vi "JSON GRUPO 1.vi"(0 "Result":cluster{u32, dbl, dbl, dbl, dbl}[](array[cluster]), 11 "error in":errorcluster) -> (4 "PAR":refnum<class "JSON Object.lvclass">[](array[class]), 6 "Humedad R.":refnum<class "JSON Object.lvclass">[](array[class]), 8 "Temp Amb":refnum<class "JSON Object.lvclass">[](array[class]), 10 "Temp Panel":refnum<class "JSON Object.lvclass">[](array[class]), 15 "error out":errorcluster)   [LabVIEW 2015]
uses:
  <vilib>/addons/JSON API/Get Polymorphic/JSON GetSet.lvlib
  <vilib>/addons/JSON API/JSON Scalar/Set SGL.vi
  <vilib>/addons/JSON API/JSON Scalar/JSON Scalar.lvclass
  <vilib>/addons/JSON API/JSON Scalar/Set U32.vi
  <vilib>/addons/JSON API/JSON Object/Set Object Item by name.vi
  <vilib>/addons/JSON API/JSON Object/JSON Object.lvclass
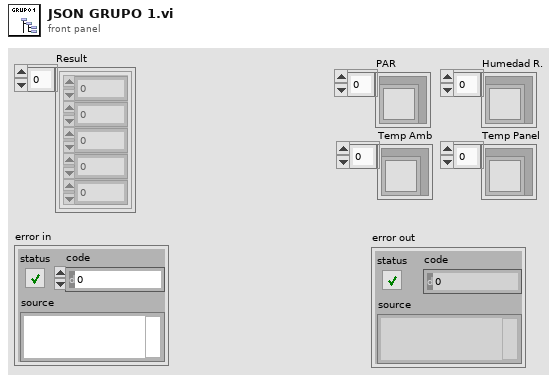
[diagram p1: front panel]
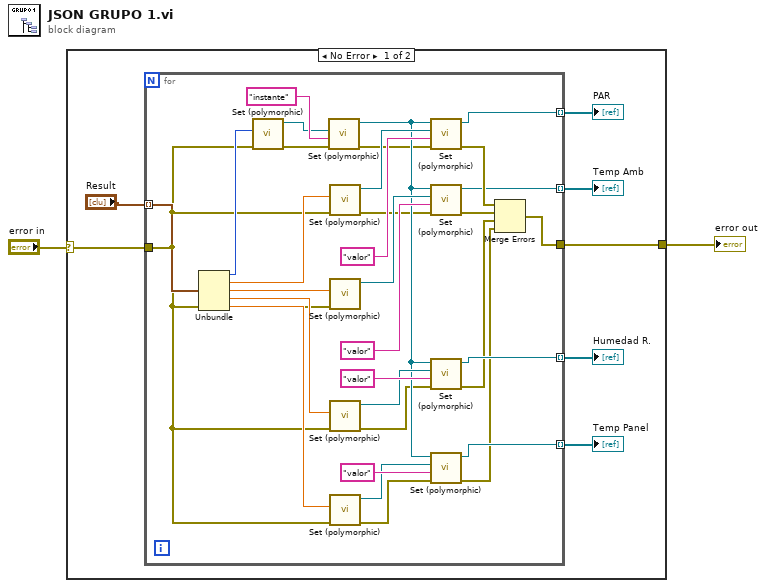
[diagram p0: block diagram]
diagram:
  n1 = case shown="No Error" "error in" {
    selector: "error in" -> [w3 w42]
    tunnel: [w8 w42] -> w1
    frame No Error {
      n2 = for {
        tunnel: "Result" -> [w41] mode=indexing
        tunnel: [w17] -> w7 mode=indexing
        tunnel: [w15] -> w6 mode=indexing
        tunnel: [w13] -> w5 mode=indexing
        tunnel: [w11] -> w4 mode=indexing
        tunnel: w3 -> [w24]
        tunnel: [w18] -> w8
        n3 = Unbundle(w41) -> (w36:u32, w40:dbl, w39:dbl, w38:dbl, w37:dbl)
        n4 = call-poly <vilib>:"Set (polymorphic).vi"("error in (no error)"=w24, "Numeric"=w36) -> ("error out"=w23:errorcluster, "JSON Scalar out"=w34:refnum<class "JSON Scalar.lvclass">)  [unwired: 8 in]
        n5 = call-poly <vilib>:"Set (polymorphic).vi"("error in (no error)"=w23, "name"="instante", "Value"=w34) -> ("error out"=w22:errorcluster, "JSON Object out"=w25:refnum<class "JSON Object.lvclass">)  [unwired: 6 in, 1 out]
        n6 = call-poly <vilib>:"Set (polymorphic).vi"("error in (no error)"=w24, "Numeric"=w40) -> ("error out"=w21:errorcluster, "JSON Scalar out"=w32:refnum<class "JSON Scalar.lvclass">)  [unwired: 8 in]
        n7 = call-poly <vilib>:"Set (polymorphic).vi"("error in (no error)"=w24, "Numeric"=w39) -> ("JSON Scalar out"=w30:refnum<class "JSON Scalar.lvclass">)  [unwired: 8 in, 1 out]
        n8 = call-poly <vilib>:"Set (polymorphic).vi"("error in (no error)"=w24, "Numeric"=w38) -> ("error out"=w20:errorcluster, "JSON Scalar out"=w28:refnum<class "JSON Scalar.lvclass">)  [unwired: 8 in]
        n9 = call-poly <vilib>:"Set (polymorphic).vi"("error in (no error)"=w24, "Numeric"=w37) -> ("error out"=w19:errorcluster, "JSON Scalar out"=w26:refnum<class "JSON Scalar.lvclass">)  [unwired: 8 in]
        n10 = call-poly <vilib>:"Set (polymorphic).vi"("error in (no error)"=w22, "name"="valor", "Value"=w32, "JSON Object in"=w25) -> ("error out"=w16:errorcluster, "JSON Object out"=w17:refnum<class "JSON Object.lvclass">)  [unwired: 5 in, 1 out]
        n11 = call-poly <vilib>:"Set (polymorphic).vi"("error in (no error)"=w21, "name"="valor", "Value"=w30, "JSON Object in"=w25) -> ("error out"=w14:errorcluster, "JSON Object out"=w15:refnum<class "JSON Object.lvclass">)  [unwired: 5 in, 1 out]
        n12 = call-poly <vilib>:"Set (polymorphic).vi"("error in (no error)"=w20, "name"="valor", "Value"=w28, "JSON Object in"=w25) -> ("error out"=w12:errorcluster, "JSON Object out"=w13:refnum<class "JSON Object.lvclass">)  [unwired: 5 in, 1 out]
        n13 = call-poly <vilib>:"Set (polymorphic).vi"("error in (no error)"=w19, "name"="valor", "Value"=w26, "JSON Object in"=w25) -> ("error out"=w10:errorcluster, "JSON Object out"=w11:refnum<class "JSON Object.lvclass">)  [unwired: 5 in, 1 out]
        n14 = Merge Errors(w16, w14, w12, w10) -> (w18:errorcluster)
      }
      "PAR" <- w7
      "Temp Amb" <- w6
      "Humedad R." <- w5
      "Temp Panel" <- w4
    }
    frame Error {
    }
  }
  "error out" <- w1
